vi "Main.vi"() -> ()   [LabVIEW 2020]
uses:
  Recog-system/Global Variables/Global Number of Indices.vi
  Recog-system/Global Variables/Global Correct Answer.vi
  Recog-system/Global Variables/Global N-Back Setting.vi
  Recog-system/Global Variables/Global User_Answer.vi
  Recog-system/Global Variables/Global Label.vi
  Recog-system/Global Variables/Training_Status.vi
  Recog-system/Global Variables/Number_of_Windows.vi
  Recog-system/Global Variables/Window_Size.vi
  Recog-system/Global Variables/Global Send To ANN.vi
  Recog-system/Global Variables/Trainning Done.vi
  Recog-system/Global Variables/Global Difficulty Level.vi
  Recog-system/Global Variables/Global Enable Logging.vi
  Recog-system/Global Variables/Global_Rating.vi
  Global Variables/Global_first_time.vi
panel:
  out "Numeric":i32
  out "Difficulty Level":u8
  out "tiggerTime":u32
  out "New square":T1
  out "seq":i8
  out "Data":bool[](array[boolean])
  out "error out":errorcluster
  out "2D Picture":picture
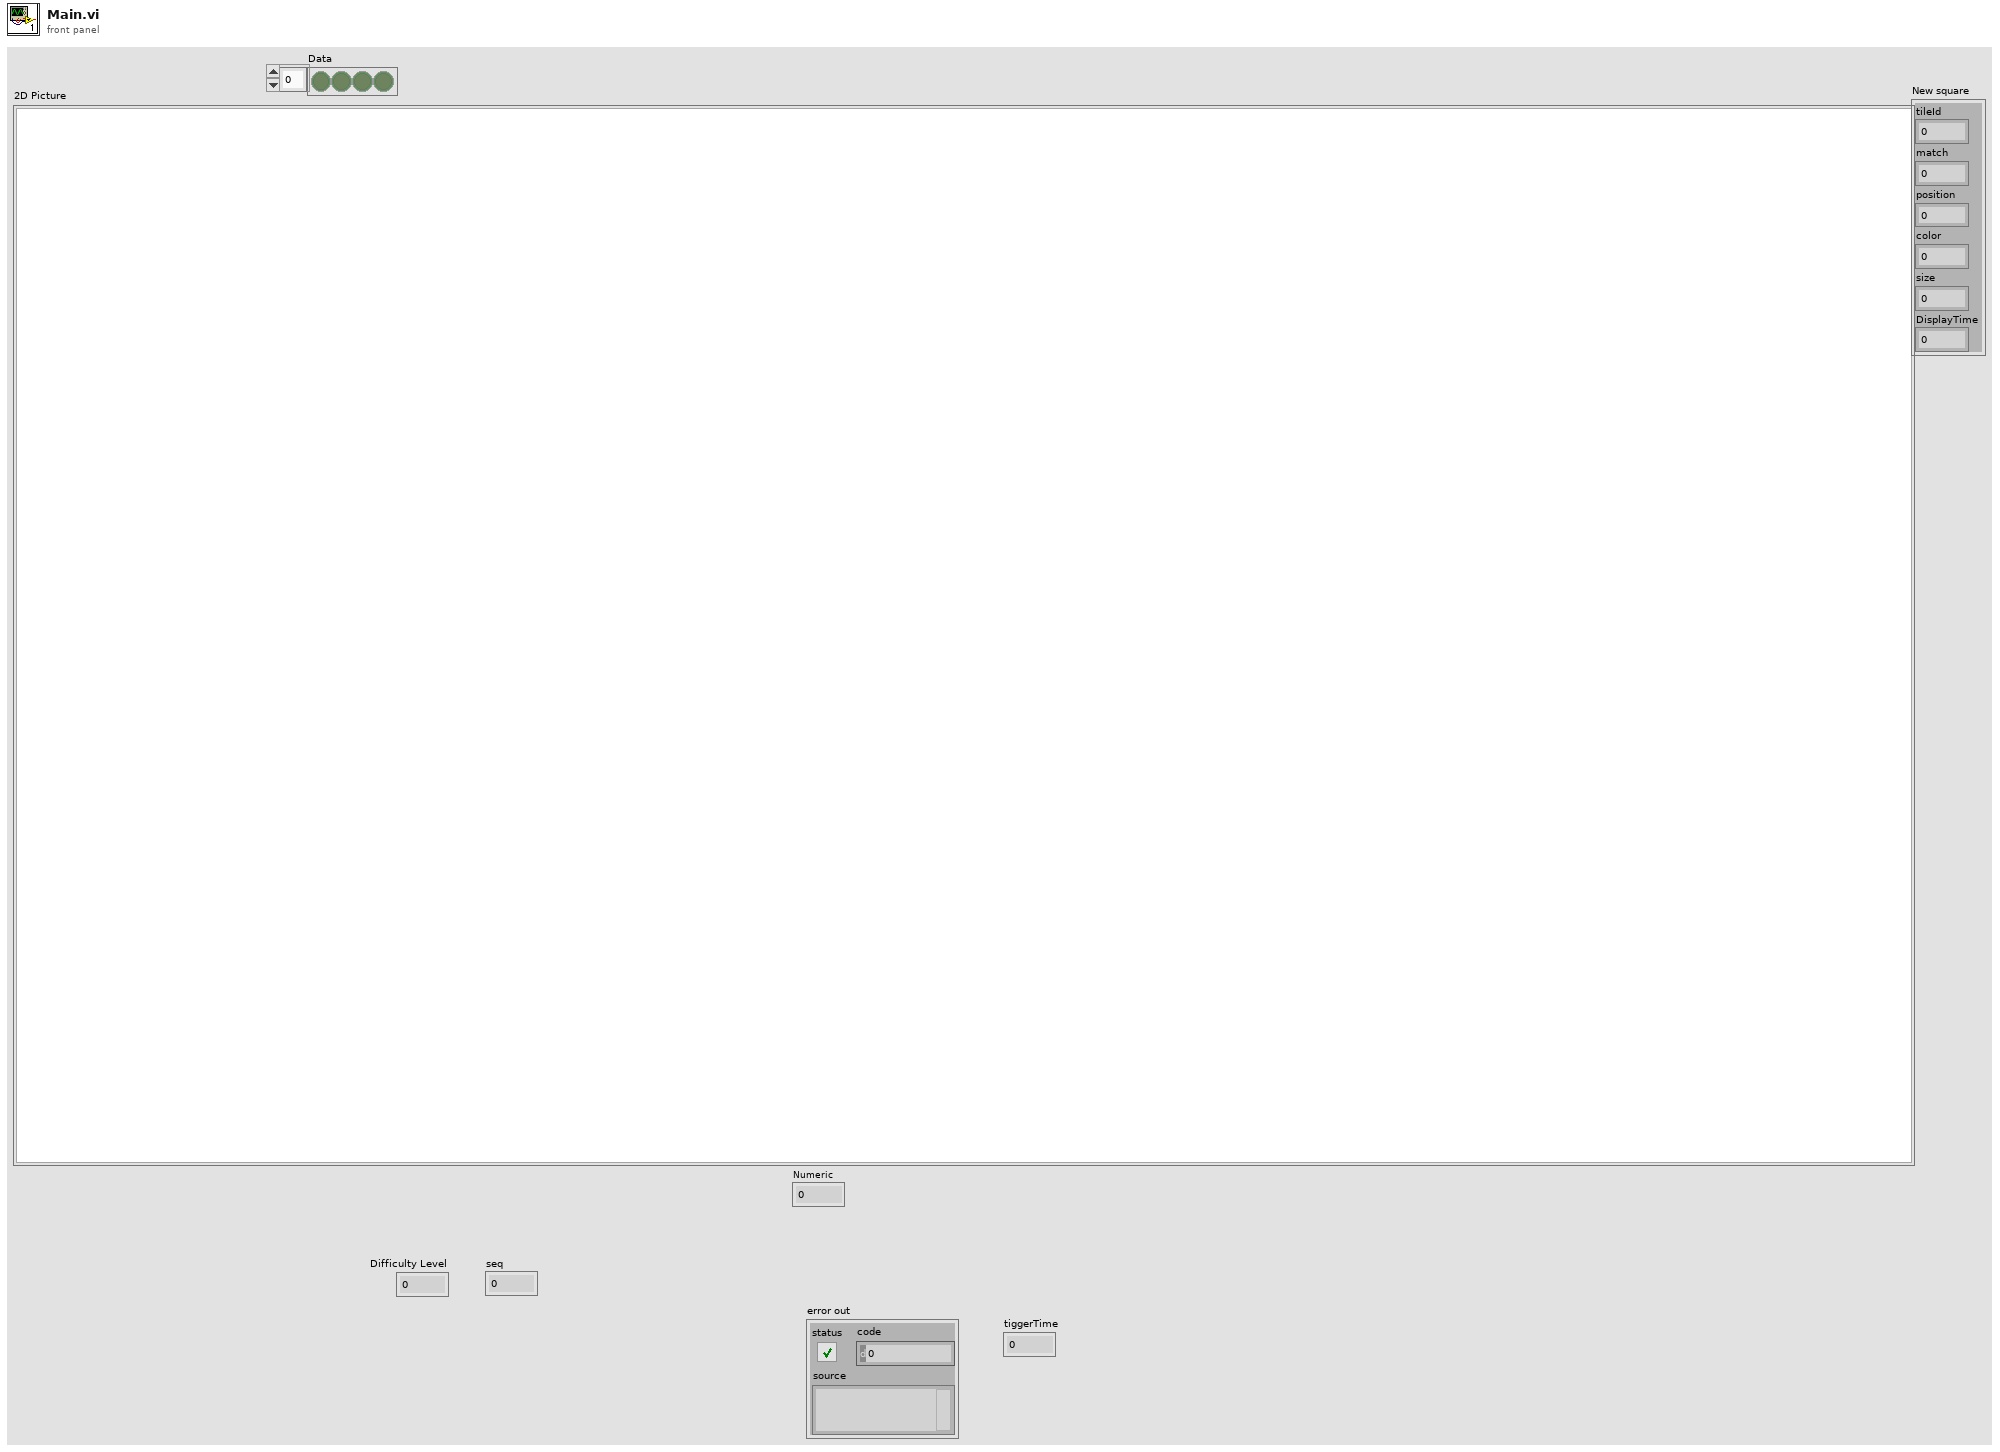
[diagram p1: front panel]
types:
  T1 = cluster{"tileId":i32, "match":i32, "position":i32, "color":u32, "size":i32, "DisplayTime":i32}
  T2 = cluster{"State":i32, "Iteration":i8, "Sequence":i8, "Counter":i8}
  T3 = cluster{"Tile size Y":dbl, "Columns":dbl, "Rows":dbl, "Cross size":dbl, "Offset X":dbl, "Tile size X":dbl, "OffsetY":dbl}
  T4 = cluster{"tileId":i32, "match":i32, "position":i32, "color":u32, "size":i32, "DisplayTime":i32}[]
  T5 = cluster{"t[0]":bool, "t[1]":bool, "t[2]":bool, "t[3]":bool, "t[4]":bool, "t[5]":bool, "t[6]":bool}
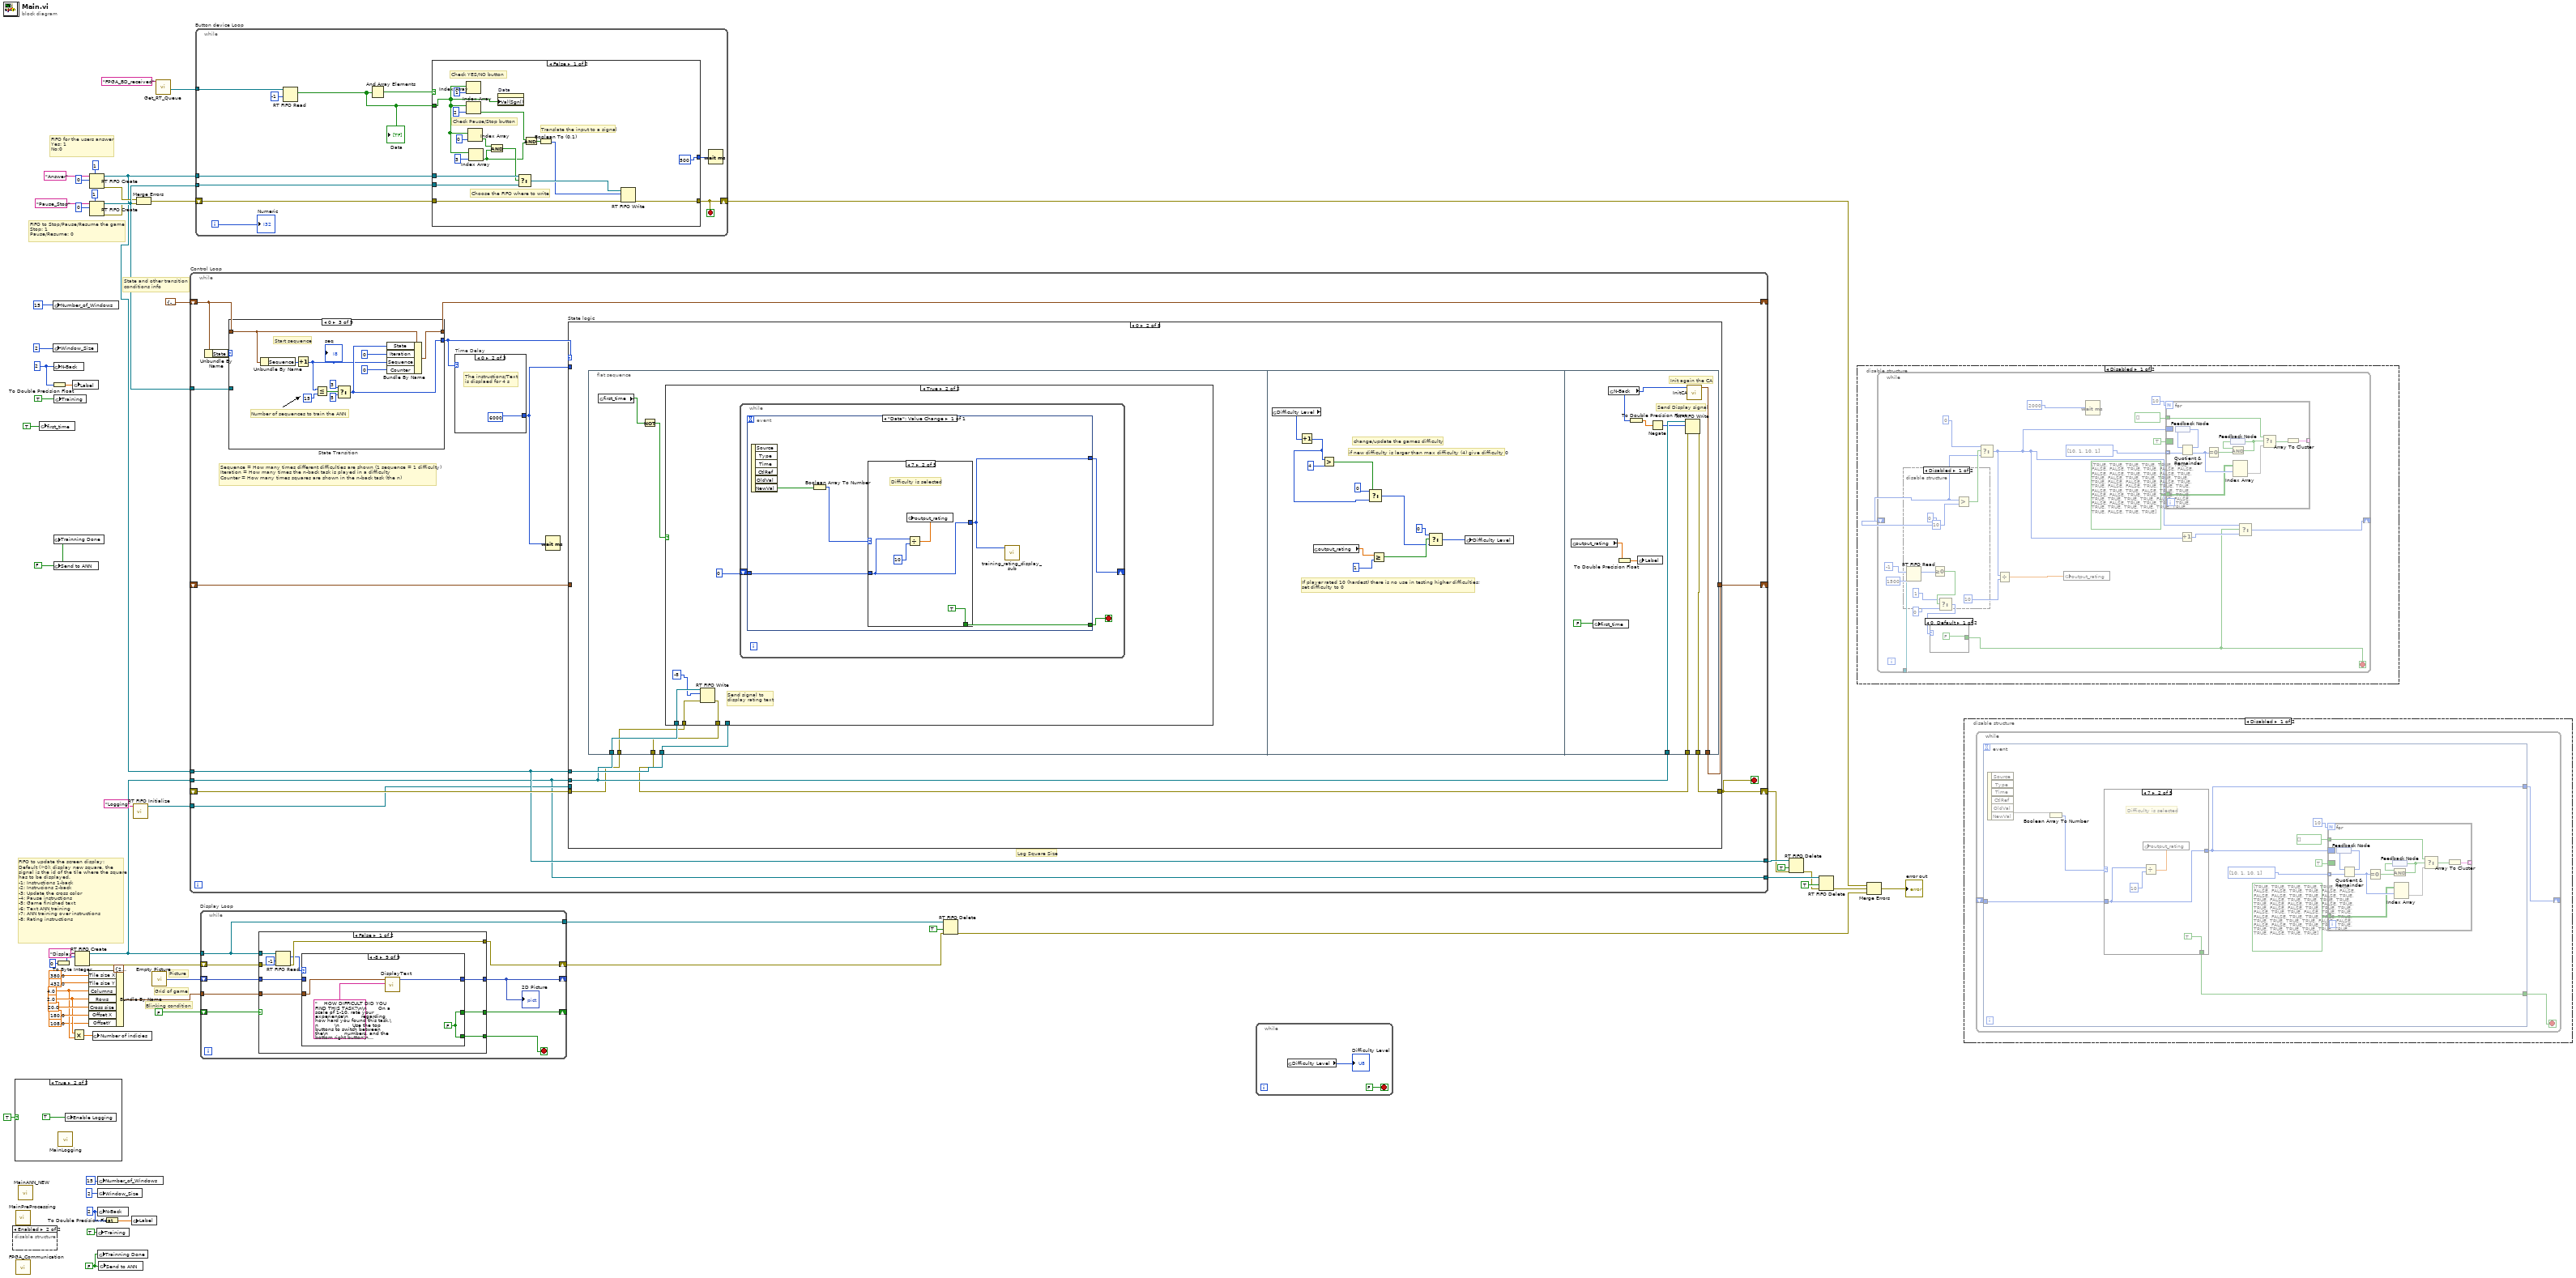
[diagram p0: block diagram]
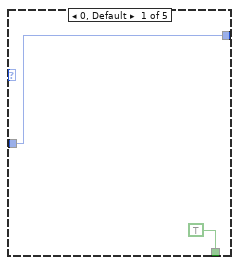
[diagram p2: hidden frame]
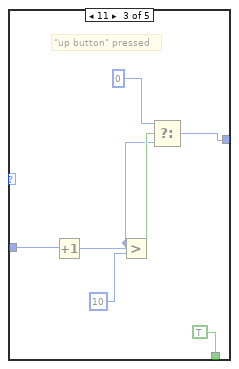
[diagram p3: hidden frame]
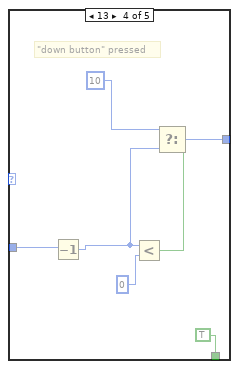
[diagram p4: hidden frame]
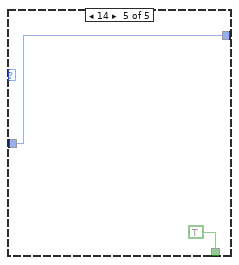
[diagram p5: hidden frame]
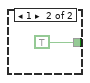
[diagram p7: hidden frame]
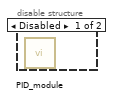
[diagram p10: hidden frame]
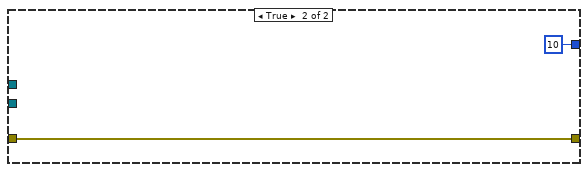
[diagram p11: hidden frame]
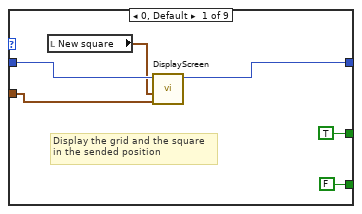
[diagram p13: hidden frame]
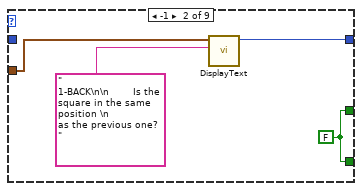
[diagram p14: hidden frame]
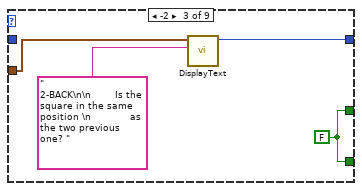
[diagram p15: hidden frame]
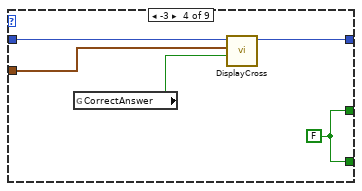
[diagram p16: hidden frame]
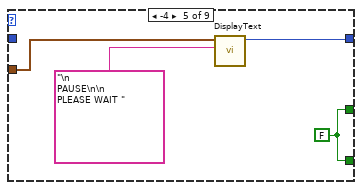
[diagram p17: hidden frame]
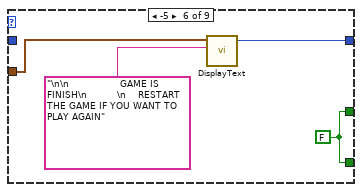
[diagram p18: hidden frame]
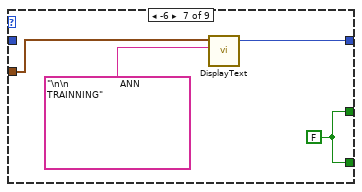
[diagram p19: hidden frame]
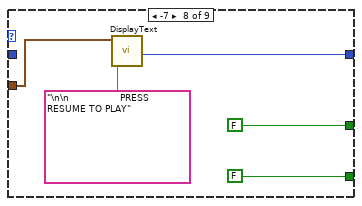
[diagram p20: hidden frame]
diagram:
  w6 = FALSE ("Send to ANN")
  w7 = u8 2 ("N-Back")
  w17 = FALSE ("Send to ANN")
  w18 = u8 2 ("N-Back")
  w47 = 2.0 ("Rows")
  w46 = 4.0 ("Columns")
  # "State and other transition \nconditions info"
  # "Picture"
  # "Grid of game"
  # "Blinking condition"
  # "FIFO to update the screen display:\nDefault (>0): display new square, the \nsignal is the id of the tile where the square\nhas to be displayed.\n-1: Instructions 1-back \n-2: Instrucions 2-back\n-3: Update the cross color \n-4: Pause instructions \n-5: Game finished text\n-6: Text ANN training\n-7: ANN training over instructions\n-8: Rating instructions"
  # "FIFO to Stop/Pause/Resume the game\nStop: 1\nPause/Resume: 0"
  # "FIFO for the users answer\nYes: 1\nNo:0"
  n1 = disable-structure shown="Enabled" {
    frame Disabled {
      n2 = call "PID_module.vi"() -> ()  [unwired: 11 in]
    }
    frame Enabled {
    }
  }
  n3 = case shown="True" TRUE {
    frame False {
    }
    frame True {
      n4 = call "MainLogging.vi"() -> ()  [unwired: 7 in]
      n5 = global write "Global Enable Logging.vi" "Enable Logging"(TRUE ("Enable Logging")) -> ()
    }
  }
  n6 = call "MainPreProcessing.vi"() -> ()  [unwired: 12 in]
  n7 = call "FPGA_Communication.vi"() -> ()  [unwired: 12 in]
  n8 = call "MainANN_NEW.vi"() -> ()  [unwired: 12 in]
  n9 = global write "Global_first_time.vi" "first_time"(TRUE ("Training")) -> ()
  n10 = To Double Precision Float(number=w18) -> (double precision float=w19:dbl)
  n11 = global write "Number_of_Windows.vi" "Number_of_Windows"(u32 15 ("Number of Windows")) -> ()
  n12 = global write "Window_Size.vi" "Window_Size"(u32 2 ("Window_Size")) -> ()
  n13 = global write "Global N-Back Setting.vi" "N-Back"(w18) -> ()
  n14 = global write "Trainning Done.vi" "Trainning Done"(w17) -> ()
  n15 = global write "Global Send To ANN.vi" "Send to ANN"(w17) -> ()
  n16 = global write "Training_Status.vi" "Training"(TRUE ("Training")) -> ()
  n17 = To Byte Integer(number=0) -> (8bit integer=w57:i8)
  n18 = Multiply(x=w47, y=w46) -> (x*y=w48:dbl)
  n19 = global write "Global Label.vi" "Label"(w19) -> ()
  n20 = RT FIFO Create(0:"Display" ("name (unnamed)"), 1:w57) -> (8:w55:refnum<k33>, 11:w37:errorcluster)  [unwired: 6 in, 1 out]
  n21 = Bundle By Name(cluster=T3 {"Tile size Y"=250.0, "Columns"=4.0, "Rows"=2.0, "Cross size"=20.0, "Offset X"=98.0, "Tile size X"=250.0, "OffsetY"=98.0} ("Grid"), "Tile size X"=380.0, "Tile size Y"=432.0 ("Tile size"), "Columns"=w46, "Rows"=w47, "Cross size"=20.0, "Offset X"=180.0 ("Offset"), "OffsetY"=108.0) -> (w36:T3)
  n22 = RT FIFO Create(0:"Answer" ("name (unnamed)"), 1:i16 0, 4:u32 1 ("size (10)")) -> (8:w2:refnum<k33>, 11:w41:errorcluster)  [unwired: 5 in, 1 out]
  n23 = RT FIFO Create(0:"Pause_Stop" ("name (unnamed)"), 1:i16 0, 4:u32 1 ("size (10)")) -> (8:w45:refnum<k33>, 11:w40:errorcluster)  [unwired: 5 in, 1 out]
  n24 = global write "Global Number of Indices.vi" "Number of indicies"(w48) -> ()
  n25 = global write "Training_Status.vi" "Training"(TRUE ("Training")) -> ()
  n26 = global write "Number_of_Windows.vi" "Number_of_Windows"(u32 15 ("Number of Windows")) -> ()
  n27 = global write "Window_Size.vi" "Window_Size"(u32 2 ("Window_Size")) -> ()
  n28 = global write "Global N-Back Setting.vi" "N-Back"(w7) -> ()
  n29 = global write "Trainning Done.vi" "Trainning Done"(w6) -> ()
  n30 = global write "Global Send To ANN.vi" "Send to ANN"(w6) -> ()
  n31 = To Double Precision Float(number=w7) -> (double precision float=w8:dbl)
  n32 = global write "Global Label.vi" "Label"(w8) -> ()
  n33 = call "RT FIFO Initialize.vi"("name (unnamed)"="Logging") -> ("rt fifo"=w13:refnum<k33>)  [unwired: 9 in, 1 out]
  n34 = Merge Errors(w41, w40) -> (w39:errorcluster)
  n35 = call "Empty Picture"() -> ("empty picture"=w53:picture)
  n36 = call "Get_RT_Queue.vi"("String"="FPGA_BD_received") -> ("rt fifo boolean"=w4:refnum<k33>)  [unwired: 8 in, 2 out]
  n37 = while "Control Loop" {
    tunnel: w55 -> [w62]
    tunnel: w2 -> [w65]
    tunnel: w45 -> [w71]
    shift-right: [w72] -> _
    shift-left: T2 {"State"=-1, "Iteration"=0, "Sequence"=0, "Counter"=0} -> [w73]
    shift-right: [w64] -> _
    shift-left: _ -> [w69]
    shift-right: [w66] -> w32
    shift-left: _ -> [w68]
    tunnel: [w65] -> w34
    tunnel: [w62] -> w33
    tunnel: w13 -> [w63]
    stop <- w66 stop-if-true
    # "Sequence = How many times different difficulties are shown (1 sequence = 1 difficulty)\nIteration = How many times the n-back task is played in a difficulty\nCounter = How many times squares are shown in the n-back task (the n)"
    # "Log Square Size"
    n38 = Unbundle By Name(w73) -> ("State"=w74:i32)
    n39 = case "State Transition" shown="0" w74 {
      tunnel: w73 -> [w277 w288 w297 w319 w332 w342 w355 w372 w383]
      tunnel: [w276 w283 w298 w318 w330 w343 w356 w371 w382] -> w72
      tunnel: w71 -> [_ _ _ w317 w328 w341 _ w373 w381]
      tunnel: [w275 0 ("f") w292 w304 w329 w339 w354 w370 w374] -> w70
      frame Default {
        w275 = -4 ("State")
        n40 = Bundle By Name(cluster=w277, "State"=w275, "Iteration"=i8 0, "Sequence"=i8 0, "Counter"=i8 0) -> (w276:T2)
      }
      frame -1 {
        # "Start state"
        n41 = Bundle By Name(cluster=w288, "State"=0, "Iteration"=i8 -1, "Sequence"=i8 0, "Counter"=i8 0) -> (w283:T2)
        n42 = global write "Global Difficulty Level.vi" "Difficulty Level"(-1) -> ()
      }
      frame 0 {
        # "Start sequence"
        # "Number of sequences to train the ANN"
        n43 = Unbundle By Name(w297) -> ("Sequence"=w296:i8)
        n44 = Increment(x=w296) -> (x+1=w290:i8)
        "seq" <- w290
        n45 = Less Or Equal?(x=w290, y=15) -> (x <= y?=w289:bool)
        n46 = Select(t=3 ("State"), s=w289, f=5) -> (s? t:f=w292:i32)
        n47 = Bundle By Name(cluster=w297, "State"=w292, "Iteration"=i8 0 ("Sequence"), "Sequence"=w290, "Counter"=i8 0) -> (w298:T2)
      }
      frame 1 {
        # "Check for Pause signal"
        # "Increase iteration number"
        # "Playing in trainning mode"
        n48 = Unbundle By Name(w319) -> ("Iteration"=w322:i8, "Sequence"=w310:i8)
        n49 = RT FIFO Read(0:w317, 1:i8 -1 ("element")) -> (9:w315:i16)  [unwired: 2 in, 4 out]
        n50 = Increment(x=w322) -> (x+1=w302:i8)
        n51 = Equal?(x=w315, y=i8 0) -> (x = y?=w312:bool)
        n52 = Less Or Equal?(x=w302, y=3) -> (x <= y?=w301:bool)
        n53 = Select(t=1 ("State"), s=w301, f=0) -> (s? t:f=w311:i32)
        n54 = Equal?(x=w310, y=12) -> (x = y?=w308:bool)
        n55 = Select(t=2, s=w312, f=w311) -> (s? t:f=w305:i32)
        n56 = Equal To 0?(x=w311) -> (x = 0?=w309:bool)
        n57 = And(x=w308, y=w309) -> (x .and. y?=w307:bool)
        n58 = Select(t=5, s=w307, f=w305) -> (s? t:f=w304:i32)
        n59 = Bundle By Name(cluster=w319, "State"=w304, "Iteration"=w302, "Sequence"=w310, "Counter"=i8 0) -> (w318:T2)
      }
      frame 2 {
        # "Waits untill it gets a Stop/Pause signal"
        # "Pause State"
        n60 = global read "Trainning Done.vi" "Trainning Done"() -> (w327:bool)
        n61 = RT FIFO Read(0:w328, 2:-1 ("timeout in ms (0)")) -> (9:w334:i16)  [unwired: 2 in, 4 out]
        n62 = Equal To 0?(x=w334) -> (x = 0?=w333:bool)
        n63 = Select(t=7, s=w327, f=3 ("timeout in ms (0)")) -> (s? t:f=w324:i32)
        n64 = Select(t=w324, s=w333, f=4) -> (s? t:f=w329:i32)
        n65 = Bundle By Name(cluster=w332, "State"=w329) -> (w330:T2)
      }
      frame 3 {
        # "State: back to normal"
        n66 = Unbundle By Name(w342) -> ("Sequence"=w350:i8, "Counter"=w340:i8)
        n67 = RT FIFO Read(0:w341, 1:i8 -1 ("element")) -> (9:w348:i16)  [unwired: 2 in, 4 out]
        n68 = Increment(x=w340) -> (x+1=w338:i8)
        n69 = Equal?(x=w348, y=i8 1) -> (x = y?=w346:bool)
        n70 = Less Or Equal?(x=w338, y=2 ("t")) -> (x <= y?=w336:bool)
        n71 = Select(t=3 ("State"), s=w336, f=1) -> (s? t:f=w345:i32)
        n72 = Select(t=2, s=w346, f=w345) -> (s? t:f=w339:i32)
        n73 = Bundle By Name(cluster=w342, "State"=w339, "Sequence"=w350, "Counter"=w338) -> (w343:T2)
      }
      frame 5 {
        # "State to wait untill the ANN is trained"
        n74 = while {
          tunnel: [w359] -> w356
          tunnel: w355 -> [w358]
          tunnel: [w357] -> w354
          stop <- w363 stop-if-true
          w357 = 6 ("State")
          n75 = global read "Trainning Done.vi" "Trainning Done"() -> (w363:bool)
          n76 = Bundle By Name(cluster=w358, "State"=w357, "Iteration"=i8 0, "Sequence"=i8 0, "Counter"=i8 0) -> (w359:T2)
        }
        n77 = Wait (ms)(milliseconds to wait=u32 1500) -> ()  [unwired: 1 out]
      }
      frame 6 {
        w370 = 7 ("s? t:f")
        # "State to wait to start to play classify"
        n78 = RT FIFO Read(0:w373, 2:-1 ("timeout in ms (0)")) -> (9:w368:i16)  [unwired: 2 in, 4 out]
        n79 = global write "Global Difficulty Level.vi" "Difficulty Level"(u8 1 ("Difficulty Level")) -> ()
        n80 = Equal To 0?(x=w368) -> (x = 0?=w367:bool)
        n81 = Select(t=7 ("timeout in ms (0)"), s=w367, f=4) -> ()  [unwired: 1 out]
        n82 = Bundle By Name(cluster=w372, "State"=w370) -> (w371:T2)
      }
      frame 7 {
        # "Check for pause signal"
        # "Playing classification"
        n83 = RT FIFO Read(0:w381, 1:i8 -1 ("element")) -> (9:w379:i16)  [unwired: 2 in, 4 out]
        n84 = Equal?(x=w379, y=i8 0) -> (x = y?=w377:bool)
        n85 = Select(t=2, s=w377, f=7) -> (s? t:f=w374:i32)
        n86 = Bundle By Name(cluster=w383, "State"=w374, "Counter"=i8 0) -> (w382:T2)
      }
    }
    n87 = case "Time Delay" shown="0" w70 {
      tunnel: [0 ("f") i64 6000 ("f") w274] -> w67
      frame Default {
      }
      frame 0 {
        # "The instructions/Text\nis displaed for 4 s"
      }
      frame 1, 3, 7 {
        n88 = call "DelayBetweenSquares.vi"() -> ("milliseconds to wait"=w274:u32)  [unwired: 10 in]
      }
    }
    n89 = Wait (ms)(milliseconds to wait=w67) -> ()  [unwired: 1 out]
    n90 = case "State logic" shown="0" w70 {
      tunnel: w62 -> [_ w79 w158 w186 w195 w222 w227 w269]
      tunnel: w65 -> [_ w80 w160 _ w197 _ _ _]
      tunnel: w69 -> [w75 _ w156 w182 w193 w219 w224 _]
      tunnel: w68 -> [w76 w77 w161 w185 w198 w221 w226 w270]
      tunnel: [w76 w81 w162 w184 w199 w220 w225 w268] -> w66
      tunnel: w67 -> [_ _ w152 _ _ _ _ _]
      tunnel: [w75 w82 w157 w182 w194 w219 w224 w266] -> w64
      tunnel: w63 -> [_ _ w149 _ w189 _ _ _]
      frame Default {
      }
      frame 0 {
        n91 = flat-sequence {
          tunnel: w80 -> [w88]
          tunnel: w79 -> [w85]
          tunnel: w77 -> [w84]
          tunnel: [w83] -> w78
          tunnel: [w144] -> w82
          tunnel: w79 -> [w142]
          tunnel: w78 -> [w140]
          tunnel: [w139] -> w81
          frame #0 {
            n92 = global read "Global_first_time.vi" "first_time"() -> (w87:bool)
            n93 = Not(x=w87) -> (.not. x?=w86:bool)
            n94 = case shown="True" w86 {
              tunnel: w88 -> [_ _]
              tunnel: w85 -> [_ w93]
              tunnel: w84 -> [w89 w92]
              tunnel: [w89 w91] -> w83
              frame False {
              }
              frame True {
                # "Send signal to \ndisplay rating text"
                n95 = RT FIFO Write(0:w93, 1:-8, 3:w92) -> (11:w91:errorcluster)  [unwired: 2 in, 3 out]
                n96 = while {
                  shift-right: [w96] -> _
                  shift-left: 0 -> [w97]
                  stop <- w95 stop-if-true
                  n97 = event shown="[0] \"Data\": Value Change" {
                    selector: _ -> [_]
                    dyn-events: _ -> [_]
                    timeout: _ -> [_]
                    tunnel: w97 -> [w100]
                    tunnel: [w99] -> w96
                    tunnel: [w98] -> w95
                    event "Data": Value Change {
                      n98 = event-data() -> ("NewVal"=w102:bool[])  [unwired: 1 in, 5 out]
                      n99 = Boolean Array To Number(Boolean array=w102) -> (number=w101:u32)
                      n100 = case shown="7" w101 {
                        tunnel: w100 -> [w103 w105 w111 w118 w123]
                        tunnel: [w103 w105 w110 w117 w123] -> w99
                        tunnel: [TRUE TRUE TRUE TRUE TRUE] -> w98
                        frame 0, Default {
                        }
                        frame 7 {
                          # "Difficulty is selected"
                          n101 = Divide(x=w105, y=10) -> (x/y=w107:dbl)
                          n102 = global write "Global_Rating.vi" "output_rating"(w107) -> ()
                        }
                        frame 11 {
                          # "\"up button\" pressed"
                          n103 = Increment(x=w111) -> (x+1=w112:i32)
                          n104 = Greater?(x=w112, y=10) -> (0:w115:bool)
                          n105 = Select(t=0, s=w115, f=w112) -> (s? t:f=w110:i32)
                        }
                        frame 13 {
                          # "\"down button\" pressed"
                          n106 = Decrement(x=w118) -> (x-1=w119:i32)
                          n107 = Less?(x=w119, y=0) -> (x < y?=w121:bool)
                          n108 = Select(t=10, s=w121, f=w119) -> (s? t:f=w117:i32)
                        }
                        frame 14 {
                        }
                      }
                      n109 = call "training_rating_display_sub.vi"("Numeric"=w99) -> ()  [unwired: 10 in, 1 out]
                    }
                  }
                }
              }
            }
          }
          frame #1 {
            # "If player rated 10 (hardest) there is no use in testing higher difficulties;\nset difficulty to 0"
            # "if new difficulty is larger than max difficulty (4) give difficulty 0"
            # "change/update the games difficulty"
            n110 = global read "Global Difficulty Level.vi" "Difficulty Level"() -> (w132:u8)
            n111 = Increment(x=w132) -> (x+1=w131:u8)
            n112 = global read "Global_Rating.vi" "output_rating"() -> (w130:dbl)
            n113 = Greater?(x=w131, y=4) -> (0:w133:bool)
            n114 = Select(t=0, s=w133, f=w131) -> (s? t:f=w127:i32)
            n115 = Greater Or Equal?(x=w130, y=1) -> (x >= y?=w128:bool)
            n116 = Select(t=0, s=w128, f=w127) -> (s? t:f=w125:i32)
            n117 = global write "Global Difficulty Level.vi" "Difficulty Level"(w125) -> ()
          }
          frame #2 {
            # "Send Display signal"
            # "Init again the CA"
            n118 = global read "Global_Rating.vi" "output_rating"() -> (w138:dbl)
            n119 = global write "Global_first_time.vi" "first_time"(FALSE) -> ()
            n120 = global read "Global N-Back Setting.vi" "N-Back"() -> (w145:u8)
            n121 = To Double Precision Float(number=w138) -> (double precision float=w137:dbl)
            n122 = To Double Precision Float(number=w145) -> (double precision float=w143:dbl)
            n123 = global write "Global Label.vi" "Label"(w137) -> ()
            n124 = Negate(x=w143) -> (-x=w141:i8)
            n125 = RT FIFO Write(0:w142, 1:w141, 3:w140) -> (11:w139:errorcluster)  [unwired: 2 in, 3 out]
            n126 = call "InitCA.vi"("N-Back"=w145) -> ("CA"=w144:T4)  [unwired: 10 in]
          }
        }
      }
      frame 1, 7 {
        # "Same logic for trainning and classify game mode"
        # "Generate new square"
        n127 = global read "Global Enable Logging.vi" "Enable Logging"() -> (w147:bool)
        n128 = call "SendTrigger.vi"("System Exe time"=200, "Window time"=0, "TimeSquares"=w152) -> ("millisecond timer value"=→"tiggerTime":u32)  [unwired: 8 in]
        n129 = call "GenerateSquare.vi"("CA"=w156) -> ("New square"=w148:T1, "Match"=w153:bool, "updated CA"=w157:T4)  [unwired: 8 in]
        n130 = case shown="True" w147 {
          tunnel: w149 -> [_ w164]
          tunnel: w148 -> [_ w163]
          frame False {
          }
          frame True {
            n131 = call "MGlogging.vi"("New square"=w163, "Refnum in"=w164) -> ()  [unwired: 9 in, 1 out]
          }
        }
        n132 = Boolean To (0,1)(Boolean=w153) -> (0, 1=w159:i16)
        n133 = flat-sequence "Check user's answer" {
          tunnel: w160 -> [w179]
          tunnel: w159 -> [w175]
          tunnel: w158 -> [w181]
          frame #0 {
            n134 = RT FIFO Read(0:w179, 1:i16 -1 ("element"), 2:1500 ("timeout in ms (0)")) -> (9:w176:i16)  [unwired: 1 in, 4 out]
            n135 = Equal?(x=w176, y=w175) -> (x = y?=w172:bool)
            n136 = Boolean To (0,1)(Boolean=w172) -> (0, 1=w174:i16)
            n137 = global write "Global Correct Answer.vi" "CorrectAnswer"(w172) -> ()
            n138 = To Single Precision Float(number=w174) -> (single precision float=w173:sgl)
            n139 = global write "Global User_Answer.vi" "Answer"(w173) -> ()
          }
          frame #1 {
            n140 = RT FIFO Write(0:w181, 1:i8 -3 ("element")) -> ()  [unwired: 3 in, 4 out]
          }
        }
        n141 = flat-sequence {
          tunnel: w158 -> [w166]
          tunnel: w161 -> [w167]
          tunnel: [w167] -> w155
          tunnel: [w166] -> w154
          tunnel: w148 -> [w165]
          tunnel: [w171] -> w162
          tunnel: w155 -> [w170]
          tunnel: w154 -> [w169]
          frame #0 {
            "New square" <- w165
          }
          frame #1 {
            n142 = RT FIFO Write(0:w169, 1:i8 0 ("element"), 3:w170) -> (11:w171:errorcluster)  [unwired: 2 in, 3 out]
          }
        }
      }
      frame 2 {
        n143 = RT FIFO Write(0:w186, 1:i8 -4 ("element"), 3:w185) -> (11:w184:errorcluster)  [unwired: 2 in, 3 out]
      }
      frame 3 {
        # "Same logic for trainning and classify game mode"
        # "Generate new square"
        n144 = global read "Global Enable Logging.vi" "Enable Logging"() -> (w187:bool)
        n145 = call "GenerateSquare.vi"("CA"=w193) -> ("New square"=w188:T1, "Match"=w190:bool, "updated CA"=w194:T4)  [unwired: 8 in]
        n146 = case shown="False" w187 {
          tunnel: w189 -> [_ w201]
          tunnel: w188 -> [_ w200]
          frame False {
          }
          frame True {
            n147 = call "MGlogging.vi"("New square"=w200, "Refnum in"=w201) -> ()  [unwired: 9 in, 1 out]
          }
        }
        n148 = Boolean To (0,1)(Boolean=w190) -> (0, 1=w196:i16)
        n149 = flat-sequence "Check user's answer" {
          tunnel: w197 -> [w216]
          tunnel: w196 -> [w212]
          tunnel: w195 -> [w218]
          frame #0 {
            w209 = TRUE ("CorrectAnswer")
            n150 = Boolean To (0,1)(Boolean=w209) -> (0, 1=w211:i16)
            n151 = global write "Global Correct Answer.vi" "CorrectAnswer"(w209) -> ()
            n152 = To Single Precision Float(number=w211) -> (single precision float=w210:sgl)
            n153 = RT FIFO Read(0:w216, 1:i16 -1 ("element"), 2:1500 ("timeout in ms (0)")) -> (9:w213:i16)  [unwired: 1 in, 4 out]
            n154 = global write "Global User_Answer.vi" "Answer"(w210) -> ()
            n155 = Equal?(x=w213, y=w212) -> ()  [unwired: 1 out]
          }
          frame #1 {
            n156 = RT FIFO Write(0:w218, 1:i8 -3 ("element")) -> ()  [unwired: 3 in, 4 out]
          }
        }
        n157 = flat-sequence {
          tunnel: w195 -> [w203]
          tunnel: w198 -> [w204]
          tunnel: [w204] -> w192
          tunnel: [w203] -> w191
          tunnel: w188 -> [w202]
          tunnel: [w208] -> w199
          tunnel: w192 -> [w207]
          tunnel: w191 -> [w206]
          frame #0 {
            n158 = local write "New square"(w202) -> ()
          }
          frame #1 {
            n159 = RT FIFO Write(0:w206, 1:i8 0 ("element"), 3:w207) -> (11:w208:errorcluster)  [unwired: 2 in, 3 out]
          }
        }
      }
      frame 4 {
        n160 = RT FIFO Write(0:w222, 1:i8 -5 ("element"), 3:w221) -> (11:w220:errorcluster)  [unwired: 2 in, 3 out]
      }
      frame 5 {
        n161 = flat-sequence {
          frame #0 {
            # "Get the rating for the last level"
            n162 = while {
              shift-right: [w231] -> _
              shift-left: 0 -> [w232]
              stop <- w230 stop-if-true
              n163 = event shown="[0]" {
                selector: _ -> [_]
                dyn-events: _ -> [_]
                timeout: _ -> [_]
                tunnel: w232 -> [w235]
                tunnel: [w234] -> w231
                tunnel: [w233] -> w230
                event [0] {
                  n164 = event-data() -> ()  [unwired: 1 in, 6 out]
                  n165 = Boolean Array To Number() -> (number=w236:u32)  [unwired: 1 in]
                  n166 = case shown="7" w236 {
                    tunnel: w235 -> [w237 w239 w245 w252 w257]
                    tunnel: [w237 w239 w244 w251 w257] -> w234
                    tunnel: [TRUE TRUE TRUE TRUE TRUE] -> w233
                    frame 0, Default {
                    }
                    frame 7 {
                      # "Difficulty is selected"
                      n167 = Divide(x=w239, y=10) -> (x/y=w241:dbl)
                      n168 = global write "Global_Rating.vi" "output_rating"(w241) -> ()
                    }
                    frame 11 {
                      # "\"up button\" pressed"
                      n169 = Increment(x=w245) -> (x+1=w246:i32)
                      n170 = Greater?(x=w246, y=10) -> (0:w249:bool)
                      n171 = Select(t=0, s=w249, f=w246) -> (s? t:f=w244:i32)
                    }
                    frame 13 {
                      # "\"down button\" pressed"
                      n172 = Decrement(x=w252) -> (x-1=w253:i32)
                      n173 = Less?(x=w253, y=0) -> (x < y?=w255:bool)
                      n174 = Select(t=10, s=w255, f=w253) -> (s? t:f=w251:i32)
                    }
                    frame 14 {
                    }
                  }
                  n175 = call "training_rating_display_sub.vi"("Numeric"=w234) -> ()  [unwired: 10 in, 1 out]
                }
              }
            }
          }
          frame #1 {
            # "Assign rating to lable"
            n176 = global read "Global_Rating.vi" "output_rating"() -> (w260:dbl)
            n177 = To Double Precision Float(number=w260) -> (double precision float=w259:dbl)
            n178 = global write "Global Label.vi" "Label"(w259) -> ()
          }
          frame #2 {
            n179 = global write "Global Send To ANN.vi" "Send to ANN"(TRUE ("Send to ANN")) -> ()
          }
          frame #3 {
            n180 = global write "Training_Status.vi" "Training"(FALSE ("Training")) -> ()
          }
          frame #4 {
            n181 = call "SendTrigger.vi"("System Exe time"=200, "Window time"=40, "TimeSquares"=1000) -> ()  [unwired: 8 in, 1 out]
          }
        }
        n182 = RT FIFO Write(0:w227, 1:i8 -6 ("element"), 3:w226) -> (11:w225:errorcluster)  [unwired: 2 in, 3 out]
      }
      frame 6 {
        # "Init the CA for the classify mode"
        n183 = global read "Global N-Back Setting.vi" "N-Back"() -> (w267:u8)
        n184 = RT FIFO Write(0:w269, 1:i8 -7 ("element"), 3:w270) -> (11:w268:errorcluster)  [unwired: 2 in, 3 out]
        n185 = call "InitCA.vi"("N-Back"=w267) -> ("CA"=w266:T4)  [unwired: 10 in]
      }
    }
  }
  n186 = while "Button device Loop" {
    tunnel: w2 -> [w394]
    tunnel: w45 -> [w393]
    shift-right: [w391] -> w28
    shift-left: w39 -> [w392]
    tunnel: w4 -> [w389]
    i -> [w386]
    stop <- w391 stop-if-true
    n187 = RT FIFO Read(0:w389, 2:-1 ("timeout in ms (0)")) -> (9:w385:bool[])  [unwired: 2 in, 4 out]
    "Data" <- w385
    n188 = And Array Elements(Boolean array=w385) -> (logical AND=w390:bool)
    n189 = case shown="False" w390 {
      tunnel: w385 -> [w395 _]
      tunnel: w394 -> [w411 _]
      tunnel: w393 -> [w410 _]
      tunnel: w392 -> [w400 w413]
      tunnel: [w399 w413] -> w391
      tunnel: [500 ("index") 10 ("index")] -> w387
      frame False {
        # "Translate the input to a signal"
        # "Choose the FIFO where to write"
        # "Check Pause/Stop button"
        # "Check YES/NO button"
        n190 = Index Array(array=w395, index=1) -> ()  [unwired: 1 out]
        n191 = Index Array(array=w395, index=2) -> (element=w404:bool)
        n192 = Index Array(array=w395, index=0) -> (element=w398:bool)
        n193 = Index Array(array=w395, index=3) -> (element=w397:bool)
        n194 = And(x=w398, y=w397) -> (x .and. y?=w405:bool)
        n195 = property on="Data" class="Arr (strict)"("Val(Sgnl)"=w395) -> ()  [unwired: 2 in, 2 out]
        n196 = Select(t=w411, s=w405, f=w410) -> (s? t:f=w402:refnum<k33>)
        n197 = And(x=w404, y=w397) -> (x .and. y?=w403:bool)
        n198 = Boolean To (0,1)(Boolean=w403) -> (0, 1=w401:i16)
        n199 = RT FIFO Write(0:w402, 1:w401, 3:w400) -> (11:w399:errorcluster)  [unwired: 2 in, 3 out]
      }
      frame True {
      }
    }
    n200 = Wait (ms)(milliseconds to wait=w387) -> ()  [unwired: 1 out]
    "Numeric" <- w386
  }
  n201 = while "Display Loop" {
    tunnel: w55 -> [w416]
    shift-right: [w421] -> _
    shift-left: FALSE -> [w422]
    shift-right: [w419] -> _
    shift-left: w53 -> [w420]
    tunnel: w36 -> [w418]
    tunnel: [w416] -> w38
    shift-right: [w414] -> w16
    shift-left: w37 -> [w415]
    stop <- w417 stop-if-true
    n202 = case shown="False" w422 {
      tunnel: [w427 FALSE] -> w421
      tunnel: w420 -> [w430 w477]
      tunnel: [w428 w476] -> w419
      tunnel: w418 -> [w429 w475]
      tunnel: w416 -> [w432 _]
      tunnel: [w426 FALSE] -> w417
      tunnel: w415 -> [w425 w473]
      tunnel: [w424 w473] -> w414
      frame False {
        n203 = RT FIFO Read(0:w432, 2:-1 ("timeout in ms (0)"), 3:w425) -> (9:w423:i8, 11:w424:errorcluster)  [unwired: 1 in, 3 out]
        n204 = case shown="-8" w423 {
          tunnel: [TRUE w440 w444 w447 w452 w456 w460 FALSE w470] -> w427
          tunnel: [w435 w442 w443 w449 w453 w457 w461 w466 w471] -> w428
          tunnel: w430 -> [w437 _ _ w450 _ _ _ _ _]
          tunnel: w429 -> [w434 w439 w446 w448 w454 w458 w462 w467 w469]
          tunnel: [FALSE w440 w444 w447 w452 w456 w460 FALSE w470] -> w426
          frame 0, Default {
            # "Display the grid and the square\nin the sended position"
            n205 = local read "New square"() -> (w433:T1)
            n206 = call "DisplayScreen.vi"("Grid"=w434, "square"=w433, "input picture"=w437) -> ("2D Picture"=w435:picture)  [unwired: 8 in]
          }
          frame -1 {
            w440 = FALSE
            n207 = call "DisplayText.vi"("text"="                      1-BACK\n\n        Is the square in the same position \n                as the previous one? ", "Grid"=w439) -> ("new picture"=w442:picture)  [unwired: 9 in]
          }
          frame -2 {
            w444 = FALSE
            n208 = call "DisplayText.vi"("text"="                      2-BACK\n\n        Is the square in the same position \n             as the two previous one? ", "Grid"=w446) -> ("new picture"=w443:picture)  [unwired: 9 in]
          }
          frame -3 {
            w447 = FALSE
            n209 = global read "Global Correct Answer.vi" "CorrectAnswer"() -> (w451:bool)
            n210 = call "DisplayCross.vi"("CorrectAnswer"=w451, "Grid"=w448, "new picture in"=w450) -> ("new picture out"=w449:picture)  [unwired: 8 in]
          }
          frame -4 {
            w452 = FALSE
            n211 = call "DisplayText.vi"("text"="\n                              PAUSE\n\n                   PLEASE WAIT ", "Grid"=w454) -> ("new picture"=w453:picture)  [unwired: 9 in]
          }
          frame -5 {
            w456 = FALSE
            n212 = call "DisplayText.vi"("text"="\n\n                 GAME IS FINISH\n          \n    RESTART THE GAME IF YOU WANT TO PLAY AGAIN", "Grid"=w458) -> ("new picture"=w457:picture)  [unwired: 9 in]
          }
          frame -6 {
            w460 = FALSE
            n213 = call "DisplayText.vi"("text"="\n\n                 ANN TRAINNING", "Grid"=w462) -> ("new picture"=w461:picture)  [unwired: 9 in]
          }
          frame -7 {
            n214 = call "DisplayText.vi"("text"="\n\n                 PRESS RESUME TO PLAY", "Grid"=w467) -> ("new picture"=w466:picture)  [unwired: 9 in]
          }
          frame -8 {
            w470 = FALSE
            n215 = call "DisplayText.vi"("text"="    HOW DIFFICULT DID YOU FIND THIS TASK?\n\n       On a scale of 1-10, rate your experience\n        regarding how hard you found this task.\n          \n        Use the top buttons to switch between the\n          numbers, and the bottom right button\n                   to confirm your answer.", "Grid"=w469) -> ("new picture"=w471:picture)  [unwired: 9 in]
          }
        }
      }
      frame True {
        # "Binking functoinality, draw the grid over the square\nto make it desapear"
        n216 = flat-sequence {
          tunnel: [w482] -> w478
          tunnel: w477 -> [w481]
          tunnel: w475 -> [w480]
          tunnel: [w483] -> w476
          tunnel: w478 -> [w483]
          frame #0 {
            n217 = call "DisplayGrid.vi"("Grid"=w480, "input picture"=w481) -> ("new picture"=w482:picture)  [unwired: 9 in]
          }
          frame #1 {
            n218 = Wait (ms)(milliseconds to wait=u32 800) -> ()  [unwired: 1 out]
          }
        }
      }
    }
    "2D Picture" <- w419
  }
  n219 = RT FIFO Delete(0:w38, 2:TRUE ("force destroy? (F)"), 3:w16) -> (11:w26:errorcluster)
  n220 = while {
    stop <- FALSE stop-if-true
    n221 = global read "Global Difficulty Level.vi" "Difficulty Level"() -> (→"Difficulty Level":u8)
  }
  n222 = RT FIFO Delete(0:w34, 2:TRUE ("force destroy? (F)"), 3:w32) -> (11:w29:errorcluster)
  n223 = RT FIFO Delete(0:w33, 2:TRUE ("force destroy? (F)"), 3:w29) -> (11:w27:errorcluster)
  n224 = disable-structure shown="Disabled" {
    frame Disabled {
      n225 = while {
        shift-right: [w496] -> _
        shift-left: 0 -> [w497]
        tunnel: _ -> [w498]
        stop <- w488 stop-if-true
        n226 = RT FIFO Read(0:w498, 1:i16 -1 ("element"), 2:1500 ("timeout in ms (0)")) -> (9:w493:i16)  [unwired: 1 in, 4 out]
        n227 = Greater Or Equal To 0?(x=w493) -> (x >= 0?=w492:bool)
        n228 = Select(t=1, s=w492, f=0) -> (s? t:f=w489:i32)
        n229 = case shown="0, Default" w489 {
          tunnel: [FALSE TRUE] -> w488
          frame 0, Default {
          }
          frame 1 {
          }
        }
        n230 = Greater?(x=w497, y=10) -> (0:w503:bool)
        n231 = Select(t=0, s=w503, f=w497) -> (s? t:f=w495:i32)
        n232 = Divide(x=w495, y=10) -> (x/y=w506:dbl)
        n233 = global write "Global_Rating.vi" "output_rating"(w506) -> ()
        n234 = Wait (ms)(milliseconds to wait=u32 2000) -> ()  [unwired: 1 out]
        n235 = for {
          N: 10 -> [_]
          border: w495 -> [_]
          tunnel: i32[] [10, 1, 10, 1] -> [w524] mode=indexing
          tunnel: [w523] -> w512 mode=indexing
          border: TRUE -> [_]
          tunnel: bool[][] [[TRUE, TRUE, TRUE, TRUE, TRUE, TRUE, FALSE], [FALSE, TRUE, TRUE, FALSE, FALSE, FALSE, FALSE], [TRUE, TRUE, FALSE, TRUE, TRUE, FALSE, TRUE], [TRUE, TRUE, TRUE, TRUE, FALSE, FALSE, TRUE], [FALSE, TRUE, TRUE, FALSE, FALSE, TRUE, TRUE], [TRUE, FALSE, TRUE, TRUE, FALSE, TRUE, TRUE], [FALSE, FALSE, TRUE, TRUE, TRUE, TRUE, TRUE], [TRUE, TRUE, TRUE, FALSE, FALSE, FALSE, FALSE], [TRUE, TRUE, TRUE, TRUE, TRUE, TRUE, TRUE], [TRUE, TRUE, TRUE, TRUE, FALSE, TRUE, TRUE]] -> [w516]
          tunnel: bool[] [] ("t") -> [w515]
          n236 = feedback #1() -> (w525:i32)
          n237 = Quotient & Remainder(x=w525, y=w524) -> (x-y*floor(x/y)=w526:i32, floor(x/y)=w522:i32)
          n238 = feedback-in #1(w526) -> ()
          n239 = Equal To 0?(x=w522) -> (x = 0?=w521:bool)
          n240 = feedback #2() -> (w520:bool)
          n241 = And(x=w520, y=w521) -> (x .and. y?=w517:bool)
          n242 = feedback-in #2(w517) -> ()
          n243 = Index Array(array=w516, index (row)=w522) -> (element=w519:bool[])  [unwired: 1 in]
          n244 = Select(t=w515, s=w517, f=w519) -> (s? t:f=w518:bool[])
          n245 = Array To Cluster(array=w518) -> (cluster=w523:T5)
        }
        n246 = Increment(x=w495) -> (x+1=w494:i32)
        n247 = Select(t=w495, s=w488, f=w494) -> (s? t:f=w496:i32)
      }
      n248 = disable-structure shown="Disabled" {
        frame Disabled {
        }
        frame Enabled {
        }
      }
    }
    frame Enabled {
    }
  }
  n249 = Merge Errors(w28, w27, w26) -> (→"error out":errorcluster)
  n250 = disable-structure shown="Disabled" {
    frame Disabled {
      n251 = while {
        shift-right: [w528] -> _
        shift-left: _ -> [w529]
        stop <- w527 stop-if-true
        n252 = event {
          selector: _ -> [_]
          dyn-events: _ -> [_]
          timeout: _ -> [_]
          tunnel: w529 -> [w532]
          tunnel: [w531] -> w528
          tunnel: [w530] -> w527
          event #0 {
            n253 = event-data() -> ("NewVal"=w540)  [unwired: 1 in, 5 out]
            n254 = Boolean Array To Number(Boolean array=w540) -> (number=w539:u32)
            n255 = case shown="7" w539 {
              tunnel: w532 -> [w553 w555 w561 w568 w573]
              tunnel: [w553 w555 w560 w567 w573] -> w531
              tunnel: [TRUE TRUE TRUE TRUE TRUE] -> w530
              frame 0, Default {
              }
              frame 7 {
                # "Difficulty is selected"
                n256 = Divide(x=w555, y=10) -> (x/y=w557:dbl)
                n257 = global write "Global_Rating.vi" "output_rating"(w557) -> ()
              }
              frame 11 {
                # "\"up button\" pressed"
                n258 = Increment(x=w561) -> (x+1=w562:i32)
                n259 = Greater?(x=w562, y=10) -> (0:w565:bool)
                n260 = Select(t=0, s=w565, f=w562) -> (s? t:f=w560:i32)
              }
              frame 13 {
                # "\"down button\" pressed"
                n261 = Decrement(x=w568) -> (x-1=w569:i32)
                n262 = Less?(x=w569, y=0) -> (x < y?=w571:bool)
                n263 = Select(t=10, s=w571, f=w569) -> (s? t:f=w567:i32)
              }
              frame 14 {
              }
            }
            n264 = for {
              N: 10 -> [_]
              border: w531 -> [_]
              tunnel: i32[] [10, 1, 10, 1] -> [w550] mode=indexing
              tunnel: [w549] -> w538 mode=indexing
              border: TRUE -> [_]
              tunnel: bool[][] [[TRUE, TRUE, TRUE, TRUE, TRUE, TRUE, FALSE], [FALSE, TRUE, TRUE, FALSE, FALSE, FALSE, FALSE], [TRUE, TRUE, FALSE, TRUE, TRUE, FALSE, TRUE], [TRUE, TRUE, TRUE, TRUE, FALSE, FALSE, TRUE], [FALSE, TRUE, TRUE, FALSE, FALSE, TRUE, TRUE], [TRUE, FALSE, TRUE, TRUE, FALSE, TRUE, TRUE], [FALSE, FALSE, TRUE, TRUE, TRUE, TRUE, TRUE], [TRUE, TRUE, TRUE, FALSE, FALSE, FALSE, FALSE], [TRUE, TRUE, TRUE, TRUE, TRUE, TRUE, TRUE], [TRUE, TRUE, TRUE, TRUE, FALSE, TRUE, TRUE]] -> [w542]
              tunnel: bool[] [] ("t") -> [w541]
              n265 = feedback #3() -> (w551:i32)
              n266 = Quotient & Remainder(x=w551, y=w550) -> (x-y*floor(x/y)=w552:i32, floor(x/y)=w548:i32)
              n267 = feedback-in #3(w552) -> ()
              n268 = Equal To 0?(x=w548) -> (x = 0?=w547:bool)
              n269 = feedback #4() -> (w546:bool)
              n270 = And(x=w546, y=w547) -> (x .and. y?=w543:bool)
              n271 = feedback-in #4(w543) -> ()
              n272 = Index Array(array=w542, index (row)=w548) -> (element=w545:bool[])  [unwired: 1 in]
              n273 = Select(t=w541, s=w543, f=w545) -> (s? t:f=w544:bool[])
              n274 = Array To Cluster(array=w544) -> (cluster=w549:T5)
            }
          }
        }
      }
    }
    frame Enabled {
    }
  }
